vi "Email_notification.vi"(0 "Email":string) -> ()   [LabVIEW 2019]
uses:
  Global/Global Variables/Data_Display_global.vi
  Instrument_Setup.vi
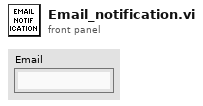
[diagram p1: front panel]
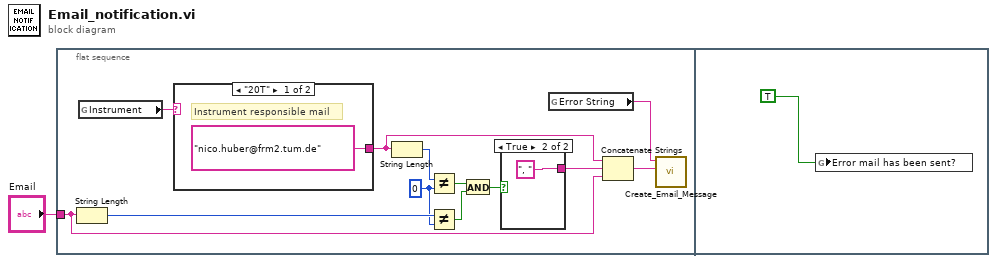
[diagram p0: block diagram]
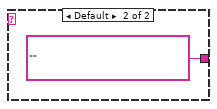
[diagram p2: hidden frame]
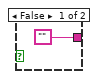
[diagram p3: hidden frame]
diagram:
  n1 = flat-sequence {
    tunnel: "Email" -> [w6]
    frame #0 {
      w5 = 0
      n2 = String Length(string=w6) -> (length=w7:i32)
      n3 = global read "Instrument_Setup.vi" "Instrument"() -> (w10:string)
      n4 = case shown="\"20T\"" w10 {
        tunnel: ["nico.huber@frm2.tum.de" ""] -> w9
        frame "20T" {
          # "Instrument responsible mail"
        }
        frame Default {
        }
      }
      n5 = String Length(string=w9) -> (length=w8:i32)
      n6 = Not Equal?(x=w8, y=w5) -> (x != y?=w4:bool)
      n7 = Not Equal?(x=w7, y=w5) -> (x != y?=w3:bool)
      n8 = And(x=w4, y=w3) -> (x .and. y?=w2:bool)
      n9 = case shown="True" w2 {
        tunnel: ["" ", "] -> w12
        frame False {
        }
        frame True {
        }
      }
      n10 = global read "Data_Display_global.vi" "Error String"() -> (w11:string)
      n11 = Concatenate Strings(w9, w12, w6) -> (w13:string)
      n12 = call "Create_Email_Message.vi"("Responsible Mail"=w13, "Warning"=w11) -> ()  [unwired: 10 in]
    }
    frame #1 {
      n13 = global write "Data_Display_global.vi" "Error mail has been sent?"(TRUE) -> ()
    }
  }
